vi "SRIMDialog.vi"(8 "Error In":errorcluster, 11 "SRIM Simulation File Path":path) -> (0 "Error Out":errorcluster, 2 "Events":dbl, 3 "SRIM Damage Peak D1 (disp * ion / cm)":dbl=nan format="%.3e")   [LabVIEW 2012]
uses:
  libs/LV-Utilities/LV-Utilities.lvlib
panel:
  in  "MOVE RIGHT":bool
  in  "MOVE LEFT":bool
  out "Events (Y)":dbl format="%.2e"
  out "D1 (X)":dbl format="%.2e"
  in  "CANCEL":bool
  in  "DONE":bool
  out "Collison Events":cluster{"Depth":dbl[], "DPA":dbl[]}(graph)
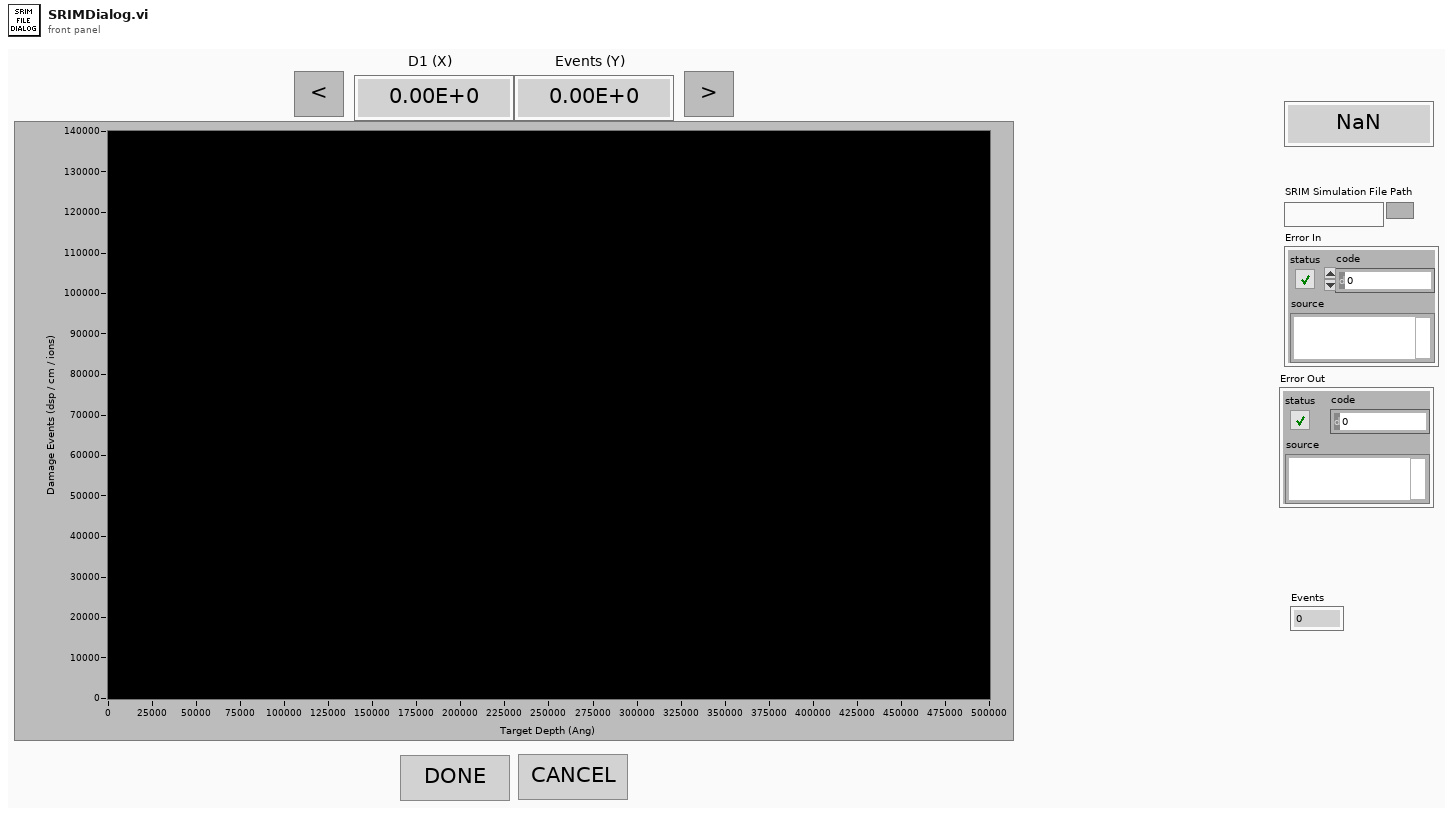
[diagram p1: front panel]
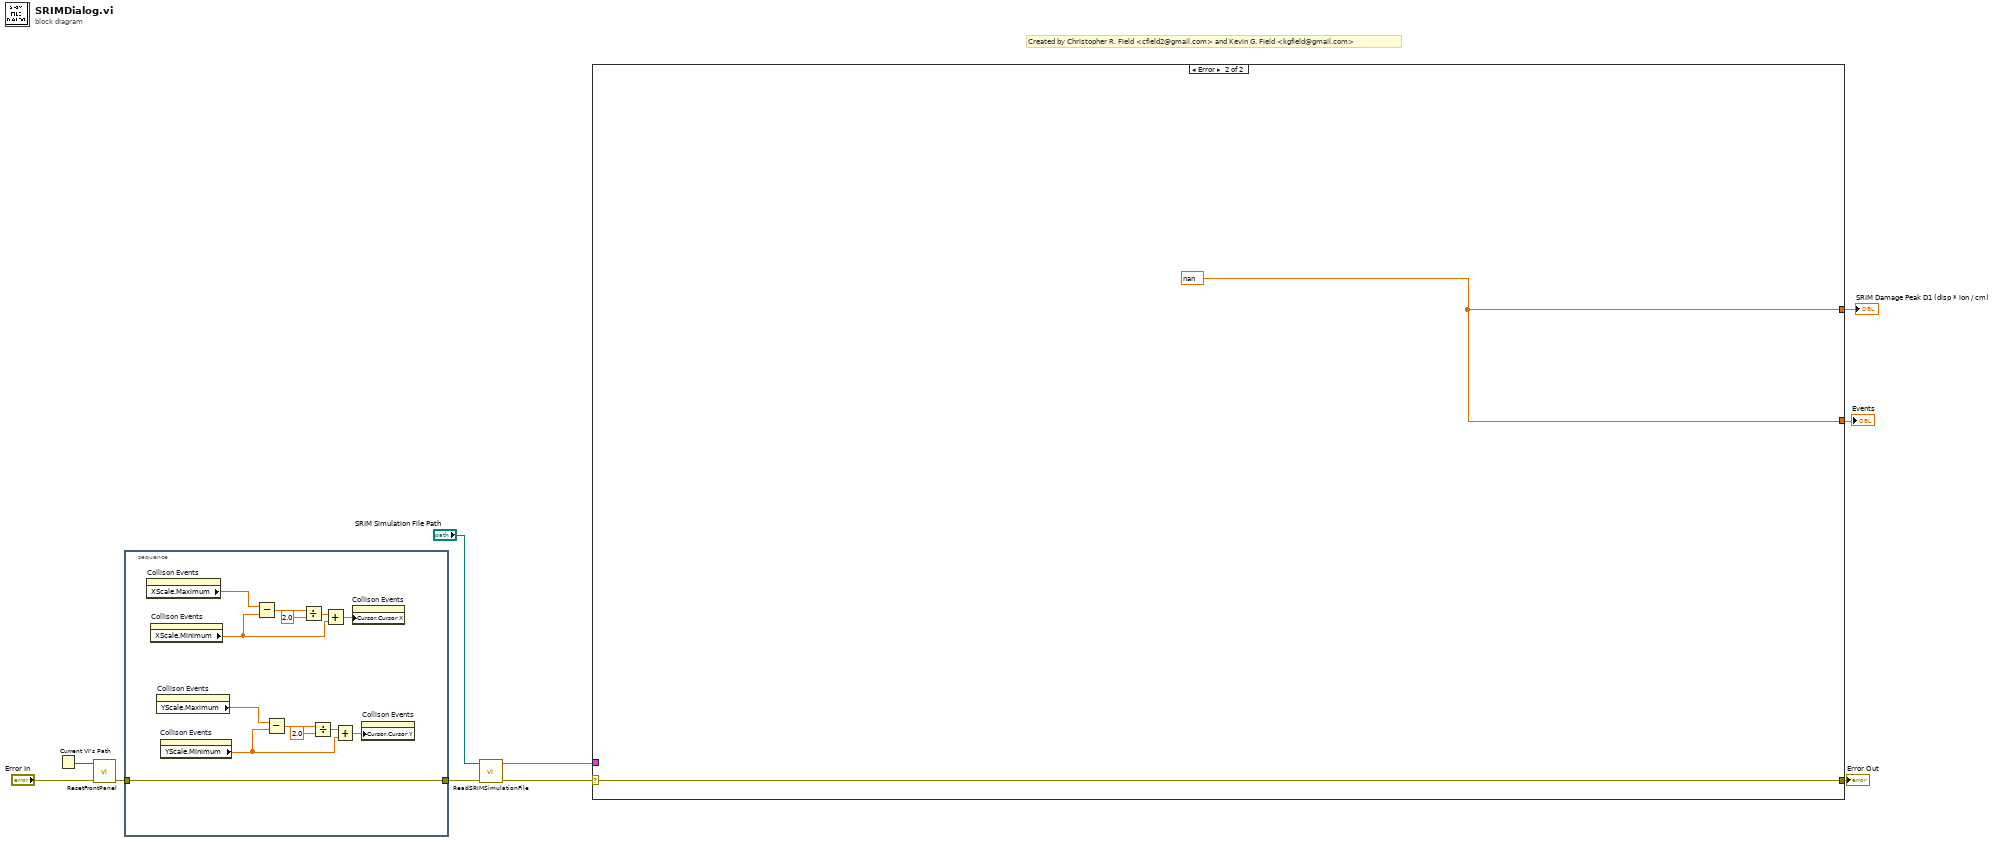
[diagram p0: block diagram]
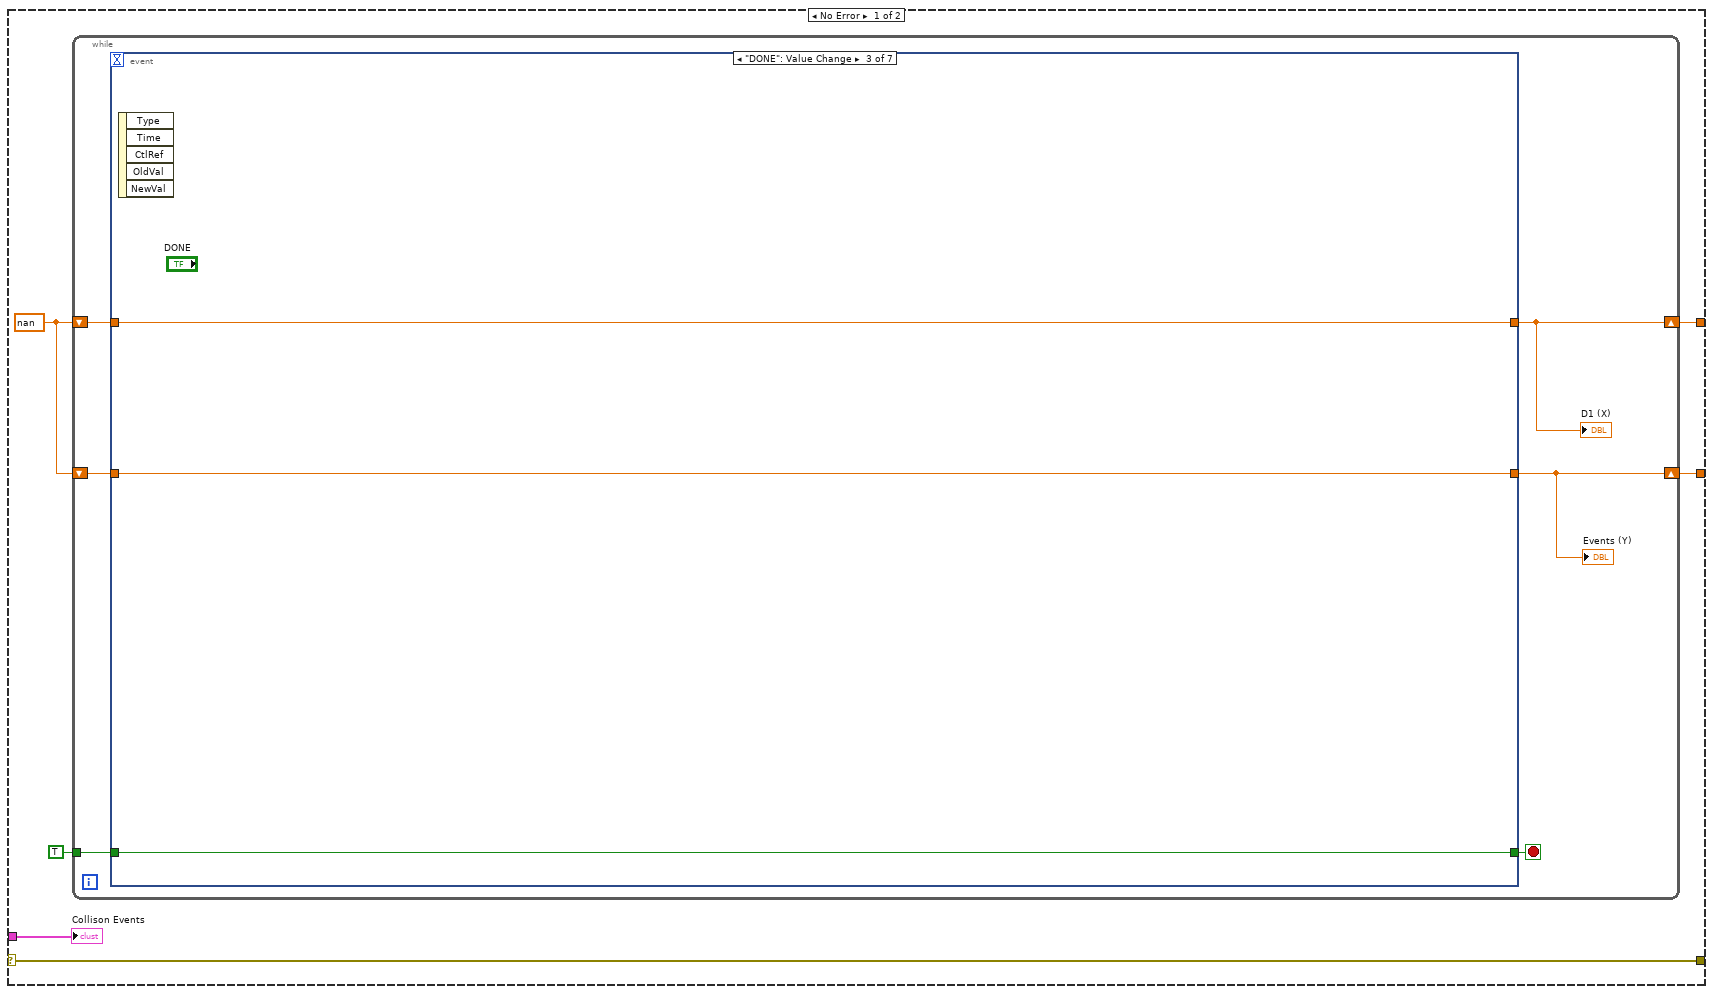
[diagram p2: hidden frame]
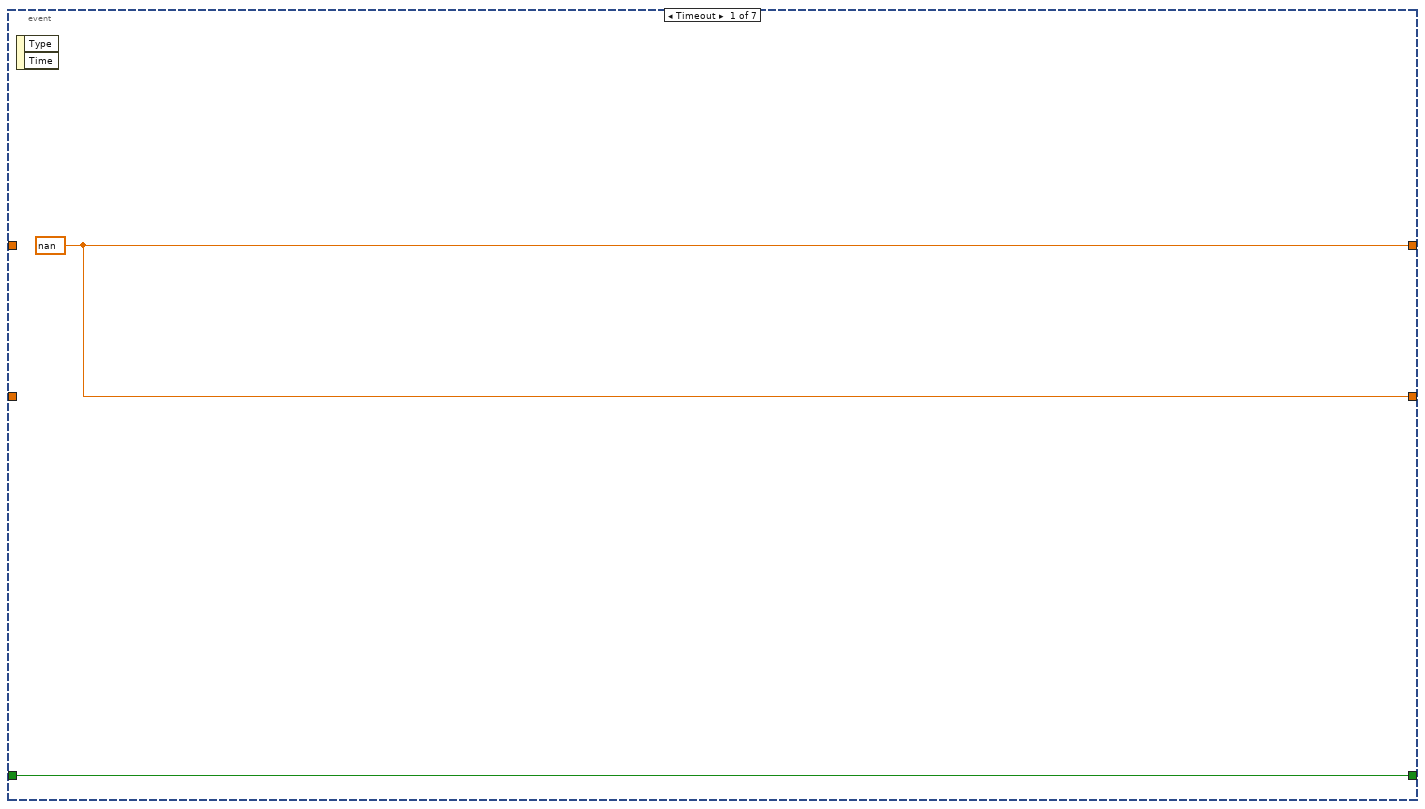
[diagram p3: hidden frame]
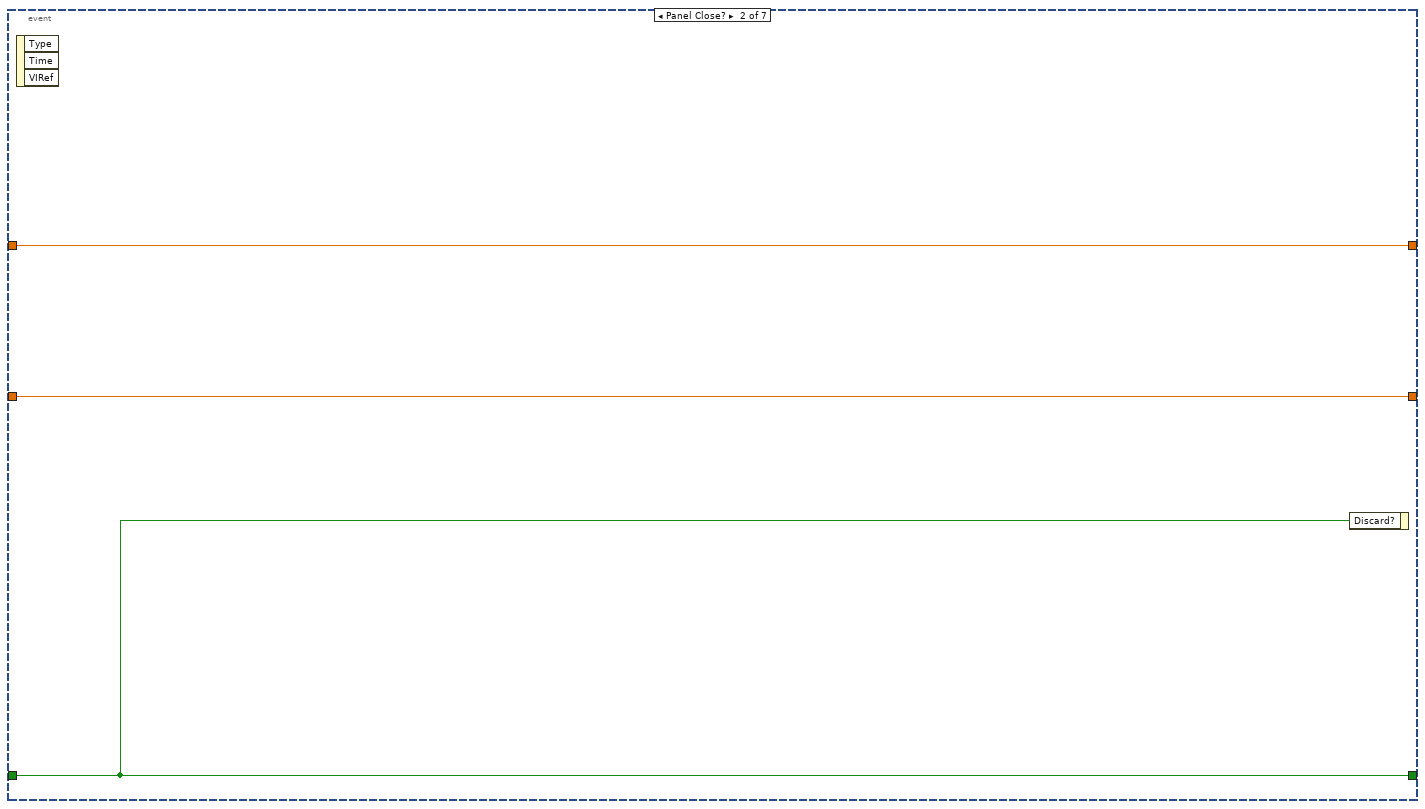
[diagram p4: hidden frame]
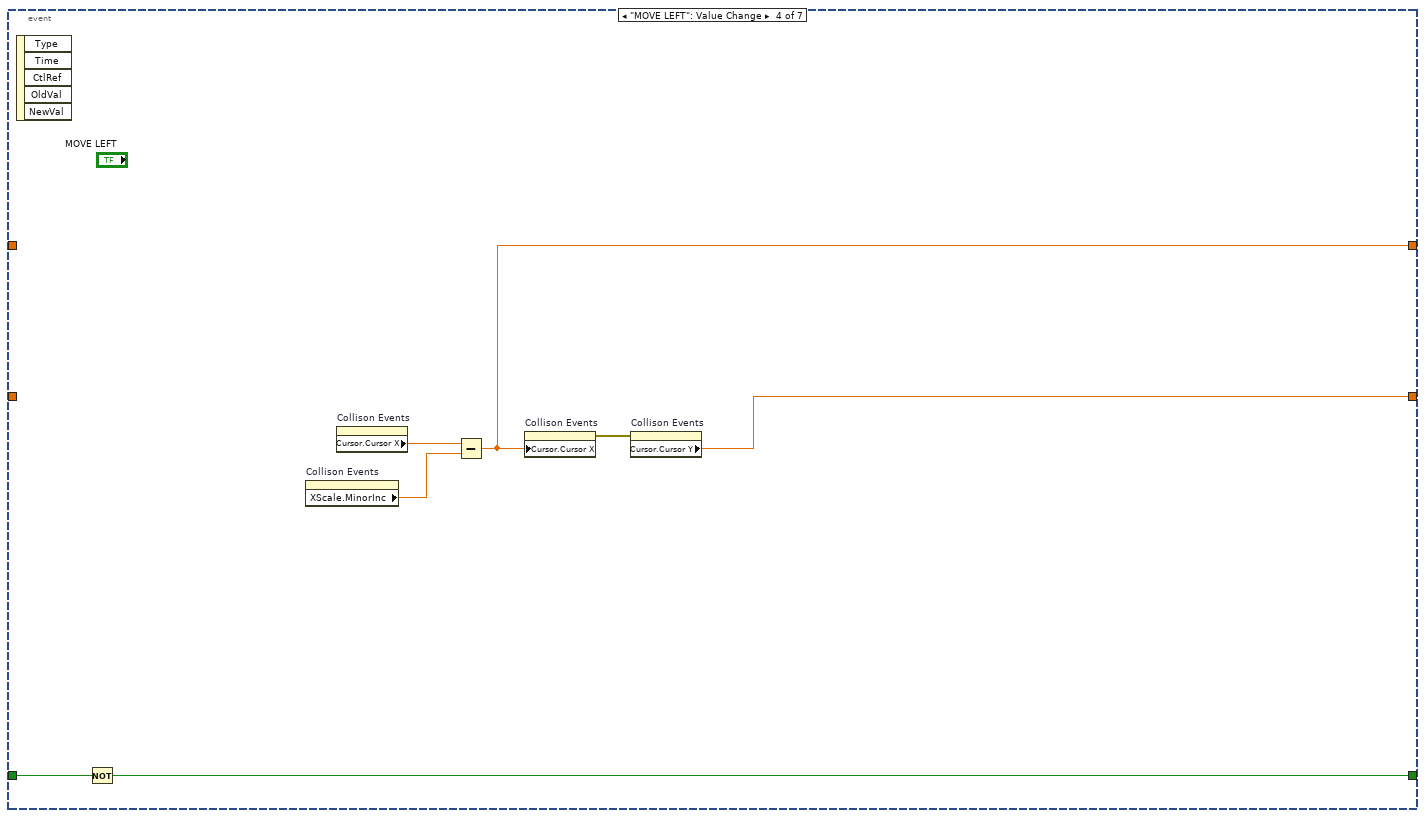
[diagram p5: hidden frame]
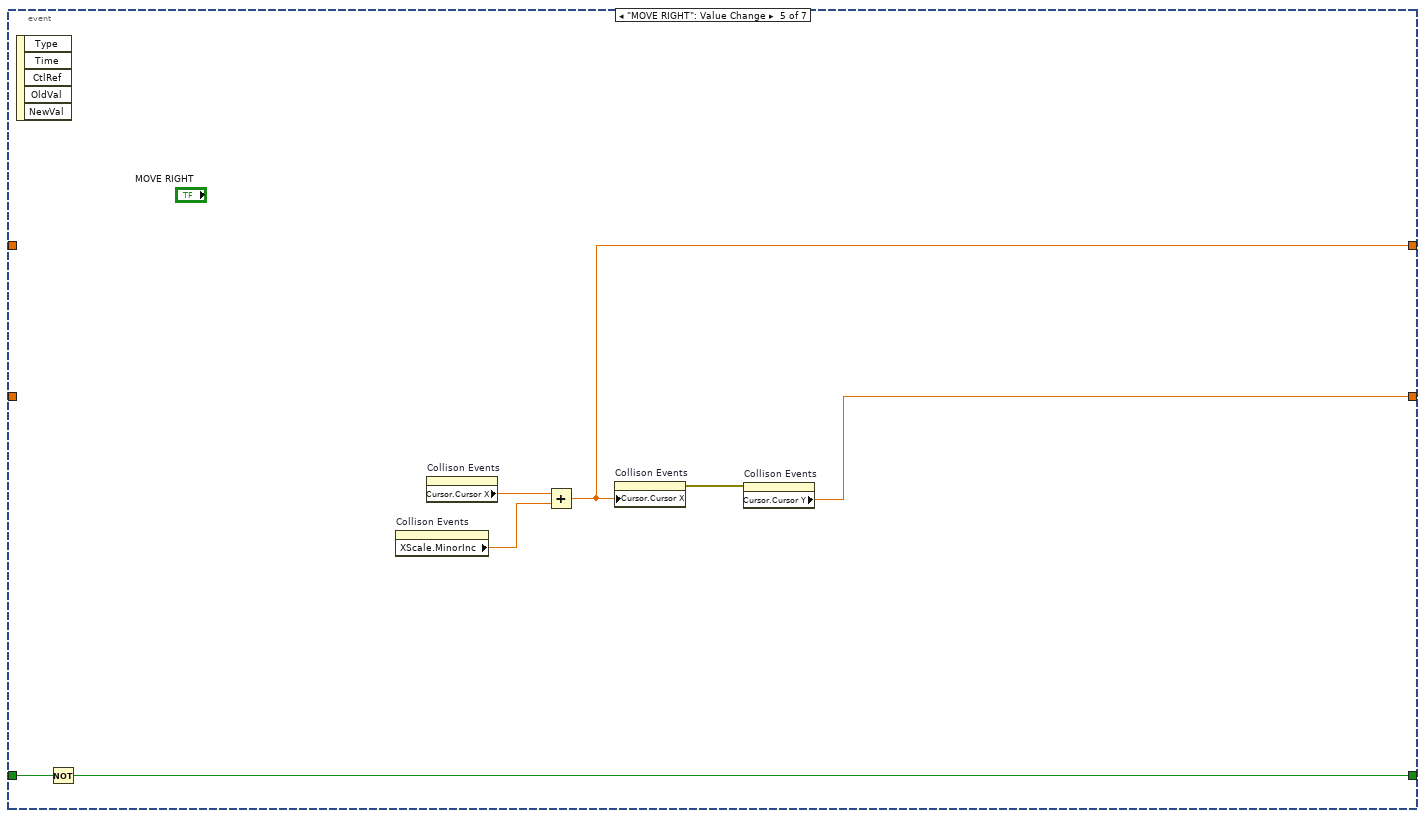
[diagram p6: hidden frame]
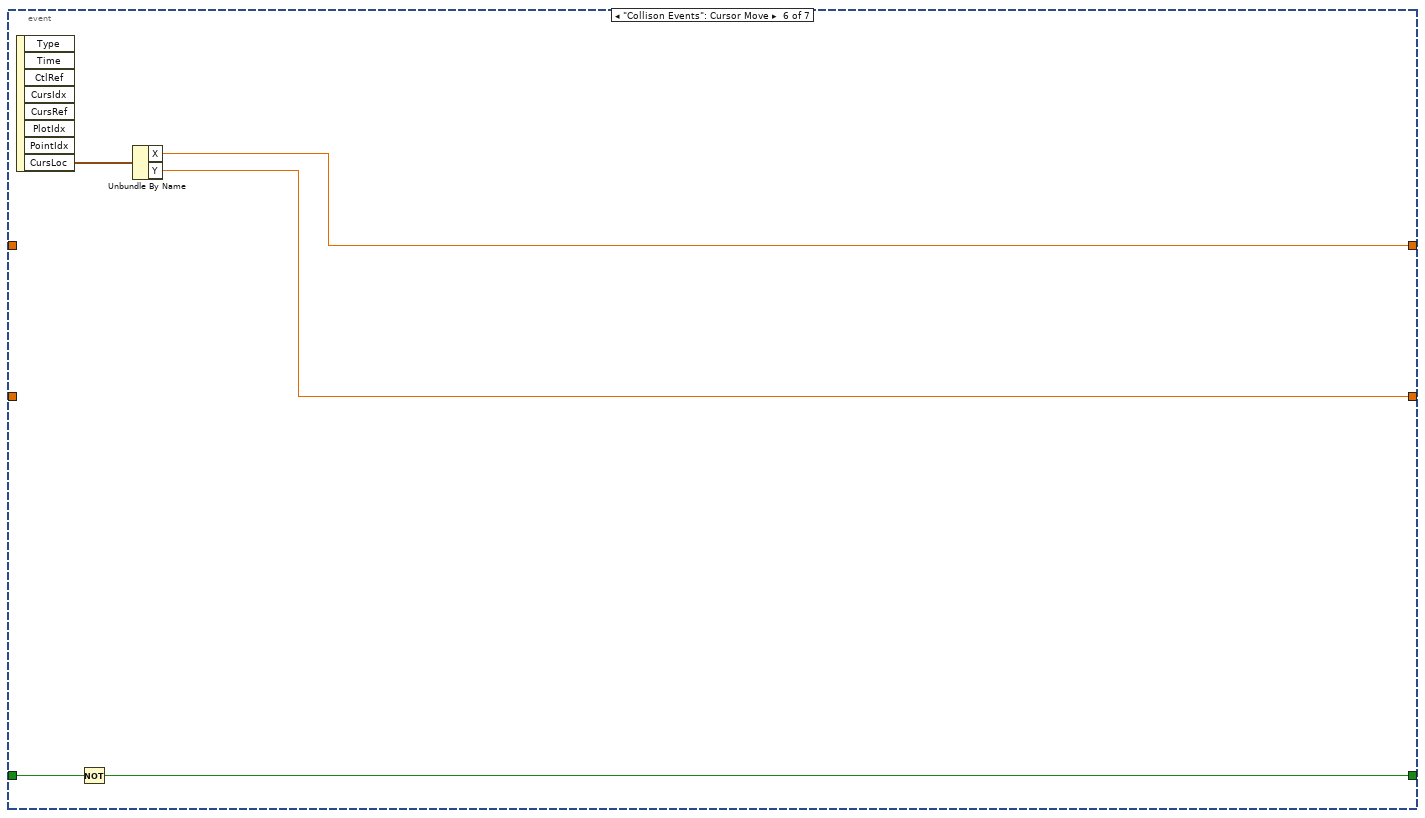
[diagram p7: hidden frame]
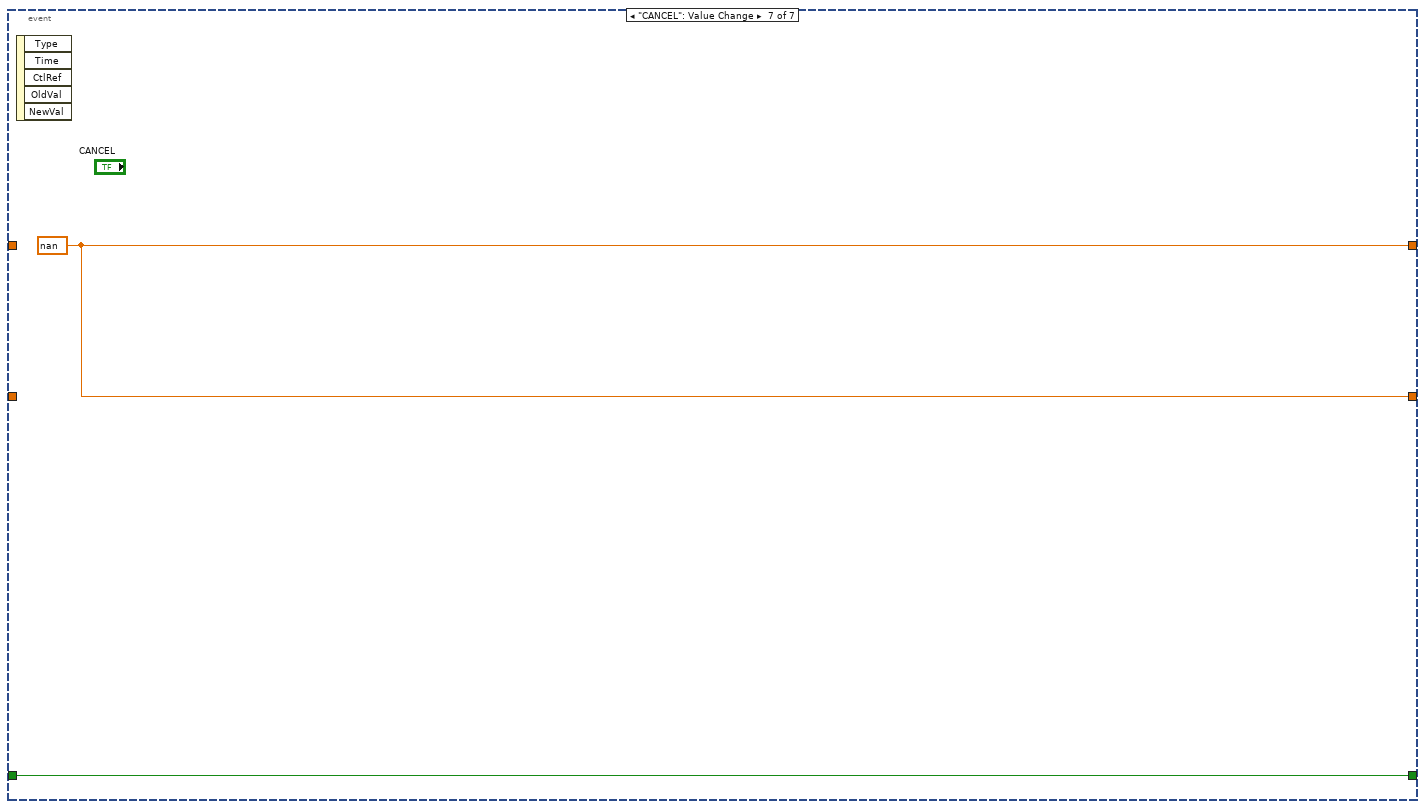
[diagram p8: hidden frame]
diagram:
  # "Created by Christopher R. Field <cfield2@gmail.com> and Kevin G. Field <kgfield@gmail.com>"
  n1 = Current VI's Path() -> (path=w7:path)
  n2 = call "ResetFrontPanel.vi"("Error In"="Error In", "VI Path"=w7) -> ("Error Out"=w3:errorcluster)  [unwired: 9 in]
  n3 = stacked-sequence {
    tunnel: w3 -> [w23]
    tunnel: [w23] -> w2
    frame #0 {
      n4 = property on="Collison Events" class="XYGraph (strict)"() -> ("XScale.Maximum"=w22:dbl)  [unwired: 2 in, 2 out]
      n5 = property on="Collison Events" class="XYGraph (strict)"() -> ("XScale.Minimum"=w18:dbl)  [unwired: 2 in, 2 out]
      n6 = property on="Collison Events" class="XYGraph (strict)"() -> ("YScale.Maximum"=w16:dbl)  [unwired: 2 in, 2 out]
      n7 = property on="Collison Events" class="XYGraph (strict)"() -> ("YScale.Minimum"=w12:dbl)  [unwired: 2 in, 2 out]
      n8 = Subtract(x=w22, y=w18) -> (x-y=w21:dbl)
      n9 = Subtract(x=w16, y=w12) -> (x-y=w15:dbl)
      n10 = Divide(x=w21, y=2.0) -> (x/y=w19:dbl)
      n11 = Divide(x=w15, y=2.0) -> (x/y=w13:dbl)
      n12 = Add(x=w19, y=w18) -> (x+y=w17:dbl)
      n13 = Add(x=w13, y=w12) -> (x+y=w11:dbl)
      n14 = property on="Collison Events" class="XYGraph (strict)"("Cursor.Cursor X"=w17) -> ()  [unwired: 2 in, 2 out]
      n15 = property on="Collison Events" class="XYGraph (strict)"("Cursor.Cursor Y"=w11) -> ()  [unwired: 2 in, 2 out]
    }
  }
  n16 = call "ReadSRIMSimulationFile.vi"("Error In"=w2, "SRIM Simulation File Path"="SRIM Simulation File Path") -> ("Error Out"=w9:errorcluster, "Collision Events"=w5:cluster{"Depth":dbl[], "DPA":dbl[]})  [unwired: 8 in]
  n17 = case shown="Error" w9 {
    selector: w9 -> [w27 w66]
    tunnel: [w28 w65] -> w10
    tunnel: [w27 w66] -> w8
    tunnel: w5 -> [w26 _]
    tunnel: [w24 w65] -> w1
    frame No Error {
      w25 = nan ("Cursor.Cursor X")
      n18 = while {
        tunnel: TRUE -> [w35]
        shift-right: [w30] -> w28
        shift-left: w25 -> [w33]
        shift-right: [w32] -> w24
        shift-left: w25 -> [w31]
        stop <- w34 stop-if-true
        n19 = event shown="[2] \"DONE\": Value Change" {
          selector: _ -> [_ _ _ _ _ _ _]
          dyn-events: _ -> [_ _ _ _ _ _ _]
          timeout: _ -> [_ _ _ _ _ _ _]
          tunnel: w35 -> [w37 w40 w43 w48 w55 w60 w64]
          tunnel: [w37 w40 w43 w47 w54 w59 w64] -> w34
          tunnel: [w36 w39 w42 w46 w53 w61 w63] -> w30
          tunnel: w33 -> [_ w39 w42 _ _ _ _]
          tunnel: [w36 w38 w41 w44 w51 w58 w63] -> w32
          tunnel: w31 -> [_ w38 w41 _ _ _ _]
          event Timeout {
            w36 = nan
            n20 = event-data() -> ()  [unwired: 1 in, 2 out]
          }
          event Panel Close? {
            n21 = event-data() -> ()  [unwired: 1 in, 3 out]
            n22 = event-data("Discard?"=w40) -> ()  [unwired: 1 in, 1 out]
          }
          event "DONE": Value Change {
            n23 = event-data() -> ()  [unwired: 1 in, 5 out]
          }
          event "MOVE LEFT": Value Change {
            n24 = event-data() -> ()  [unwired: 1 in, 5 out]
            n25 = Not(x=w48) -> (.not. x?=w47:bool)
            n26 = property on="Collison Events" class="XYGraph (strict)"() -> ("XScale.MinorInc"=w49:dbl)  [unwired: 2 in, 2 out]
            n27 = property on="Collison Events" class="XYGraph (strict)"() -> ("Cursor.Cursor X"=w50:dbl)  [unwired: 2 in, 2 out]
            n28 = Subtract(x=w50, y=w49) -> (x-y=w46:dbl)
            n29 = property on="Collison Events" class="XYGraph (strict)"("Cursor.Cursor X"=w46) -> (error out=w45:errorcluster)  [unwired: 2 in, 1 out]
            n30 = property on="Collison Events" class="XYGraph (strict)"(error in=w45) -> ("Cursor.Cursor Y"=w44:dbl)  [unwired: 1 in, 2 out]
          }
          event "MOVE RIGHT": Value Change {
            n31 = event-data() -> ()  [unwired: 1 in, 5 out]
            n32 = Not(x=w55) -> (.not. x?=w54:bool)
            n33 = property on="Collison Events" class="XYGraph (strict)"() -> ("XScale.MinorInc"=w56:dbl)  [unwired: 2 in, 2 out]
            n34 = property on="Collison Events" class="XYGraph (strict)"() -> ("Cursor.Cursor X"=w57:dbl)  [unwired: 2 in, 2 out]
            n35 = Add(x=w57, y=w56) -> (x+y=w53:dbl)
            n36 = property on="Collison Events" class="XYGraph (strict)"("Cursor.Cursor X"=w53) -> (error out=w52:errorcluster)  [unwired: 2 in, 1 out]
            n37 = property on="Collison Events" class="XYGraph (strict)"(error in=w52) -> ("Cursor.Cursor Y"=w51:dbl)  [unwired: 1 in, 2 out]
          }
          event "Collison Events": Cursor Move {
            n38 = event-data() -> ("CursLoc"=w62:cluster{"X":dbl, "Y":dbl})  [unwired: 1 in, 7 out]
            n39 = Not(x=w60) -> (.not. x?=w59:bool)
            n40 = Unbundle By Name(w62) -> ("X"=w61:dbl, "Y"=w58:dbl)
          }
          event "CANCEL": Value Change {
            w63 = nan
            n41 = event-data() -> ()  [unwired: 1 in, 5 out]
          }
        }
        "D1 (X)" <- w30
        "Events (Y)" <- w32
      }
      "Collison Events" <- w26
    }
    frame Error {
      w65 = nan ("Cursor.Cursor X")
    }
  }
  "SRIM Damage Peak D1 (disp * ion / cm)" <- w10
  "Error Out" <- w8
  "Events" <- w1
